vi "Read Objects.vi"(8 "error in":errorcluster, 11 "device data model in":refnum<class "Standard Data Model.lvclass">) -> (0 "error out":errorcluster, 2 "Objects":T1[](array[typedef]) {"Object ID" format="%x"}, 3 "device data model out":refnum<class "Standard Data Model.lvclass">)   [LabVIEW 2012, in "Standard Data Model.lvclass"]
doc: "Retrieves objects from the device model."
uses:
  Standard Data Model.lvclass
  Identification Parameters.ctl
  Standard Data Model.lvclass/Standard Data Model.ctl
  Device Data Model.lvclass
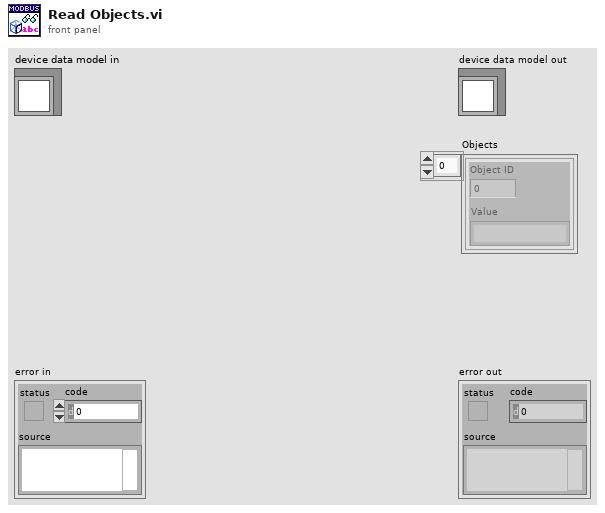
[diagram p1: front panel]
types:
  T1 = typedef "Device Data Model.lvclass/Identification Parameters.ctl" = cluster{"Object ID":u8, "Value":string}
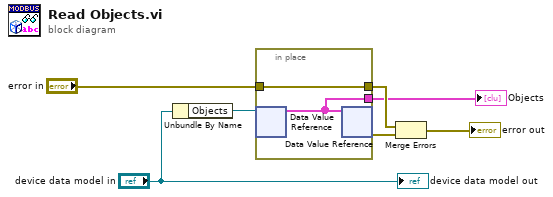
[diagram p0: block diagram]
diagram:
  n1 = Unbundle By Name("device data model in") -> ("Objects"=w5:refnum<data-value>)
  n2 = in-place {
    in-place-border: "error in" -> [w9]
    in-place-border: [w9] -> w2
    in-place-border: [w8] -> w1
    n3 = in-place-dvr #1(w5) -> (w8:T1[])  [unwired: 1 out]
    n4 = in-place-dvr #1(w8) -> (w3:errorcluster)  [unwired: 1 out]
  }
  "Objects" <- w1
  n5 = Merge Errors(w2, w3) -> (→"error out":errorcluster)
  "device data model out" <- "device data model in"
